vi "Test Packet Identifier.vi"() -> ()   [LabVIEW 2013]
uses:
  Control Packets/CONNECT/CONNECT.lvclass
  Control Packets/CONNACK/CONNACK.lvclass
  Control Packets/PUBLISH/PUBLISH.lvclass
  Control Packets/PUBACK/PUBACK.lvclass
  Control Packets/PUBREC/PUBREC.lvclass
  Control Packets/PUBREL/PUBREL.lvclass
  Control Packets/PUBCOMP/PUBCOMP.lvclass
  Control Packets/SUBSCRIBE/SUBSCRIBE.lvclass
  Control Packets/SUBACK/SUBACK.lvclass
  Control Packets/UNSUBSCRIBE/UNSUBSCRIBE.lvclass
  Control Packets/UNSUBACK/UNSUBACK.lvclass
  Control Packets/PINGREC/PINGREC.lvclass
  Control Packets/PINGRESP/PINGRESP.lvclass
  Control Packets/DISCONNECT/DISCONNECT.lvclass
  Control Packets/ControlPacket/ControlPacket.lvclass/ControlPacket.ctl
  Control Packets/ControlPacket/ControlPacket.lvclass
panel:
  out "PASS":bool
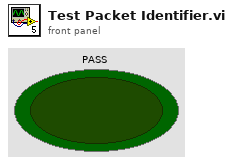
[diagram p1: front panel]
types:
  T1 = cluster{"CONNECT":refnum<class "CONNECT.lvclass">, "CONNACK":refnum<class "CONNACK.lvclass">, "PUBLISH":refnum<class "PUBLISH.lvclass">, "PUBACK":refnum<class "PUBACK.lvclass">, "PUBREC":refnum<class "PUBREC.lvclass">, "PUBREL":refnum<class "PUBREL.lvclass">, "PUBCOMP":refnum<class "PUBCOMP.lvclass">, "SUBSCRIBE":refnum<class "SUBSCRIBE.lvclass">, "SUBACK":refnum<class "SUBACK.lvclass">, "UNSUBSCRIBE":refnum<class "UNSUBSCRIBE.lvclass">, "UNSUBACK":refnum<class "UNSUBACK.lvclass">, "PINGREC":refnum<class "PINGREC.lvclass">, "PINGRESP":refnum<class "PINGRESP.lvclass">, "DISCONNECT":refnum<class "DISCONNECT.lvclass">}
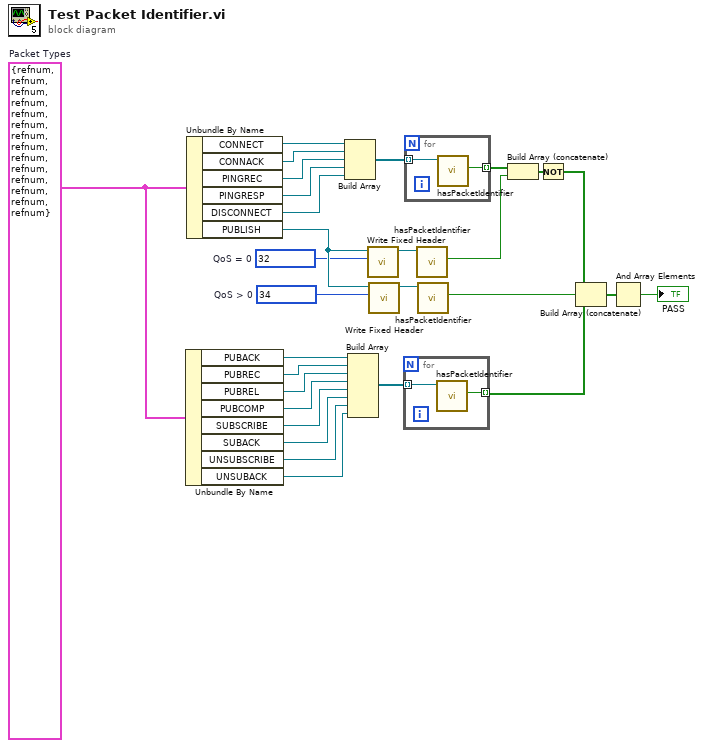
[diagram p0: block diagram]
diagram:
  w1 = u8 32  # QoS = 0
  w11 = u8 34  # QoS > 0
  w29 = T1 {"CONNECT"=refnum, "CONNACK"=refnum, "PUBLISH"=refnum, "PUBACK"=refnum, "PUBREC"=refnum, "PUBREL"=refnum, "PUBCOMP"=refnum, "SUBSCRIBE"=refnum, "SUBACK"=refnum, "UNSUBSCRIBE"=refnum, "UNSUBACK"=refnum, "PINGREC"=refnum, "PINGRESP"=refnum, "DISCONNECT"=refnum}  # Packet Types
  n1 = Unbundle By Name(w29) -> ("PUBACK"=w23:refnum<class "PUBACK.lvclass">, "PUBREC"=w22:refnum<class "PUBREC.lvclass">, "PUBREL"=w21:refnum<class "PUBREL.lvclass">, "PUBCOMP"=w20:refnum<class "PUBCOMP.lvclass">, "SUBSCRIBE"=w19:refnum<class "SUBSCRIBE.lvclass">, "SUBACK"=w18:refnum<class "SUBACK.lvclass">, "UNSUBSCRIBE"=w17:refnum<class "UNSUBSCRIBE.lvclass">, "UNSUBACK"=w16:refnum<class "UNSUBACK.lvclass">)
  n2 = Unbundle By Name(w29) -> ("CONNECT"=w28:refnum<class "CONNECT.lvclass">, "CONNACK"=w27:refnum<class "CONNACK.lvclass">, "PINGREC"=w26:refnum<class "PINGREC.lvclass">, "PINGRESP"=w25:refnum<class "PINGRESP.lvclass">, "DISCONNECT"=w24:refnum<class "DISCONNECT.lvclass">, "PUBLISH"=w3:refnum<class "PUBLISH.lvclass">)
  n3 = Build Array(w28, w27, w26, w25, w24) -> (w15:refnum<class "ControlPacket.lvclass">[])
  n4 = Build Array(w23, w22, w21, w20, w19, w18, w17, w16) -> (w14:refnum<class "ControlPacket.lvclass">[])
  n5 = call "Write Fixed Header.vi"("Fixed Header"=w1, "ControlPacket in"=w3) -> ("ControlPacket out"=w2:refnum<class "PUBLISH.lvclass">)  [unwired: 9 in]
  n6 = call "Write Fixed Header.vi"("Fixed Header"=w11, "ControlPacket in"=w3) -> ("ControlPacket out"=w10:refnum<class "PUBLISH.lvclass">)  [unwired: 9 in]
  n7 = for {
    tunnel: w14 -> [w31] mode=indexing
    tunnel: [w30] -> w8 mode=indexing
    n8 = call-dynamic "hasPacketIdentifier.vi"("ControlPacket in"=w31) -> ("As Packet Identifier"=w30:bool)  [unwired: 9 in, 1 out]
  }
  n9 = for {
    tunnel: w15 -> [w33] mode=indexing
    tunnel: [w32] -> w7 mode=indexing
    n10 = call-dynamic "hasPacketIdentifier.vi"("ControlPacket in"=w33) -> ("As Packet Identifier"=w32:bool)  [unwired: 9 in, 1 out]
  }
  n11 = call-dynamic "hasPacketIdentifier.vi"("PUBLISH in"=w2) -> ("As Packet Identifier"=w6:bool)  [unwired: 9 in, 1 out]
  n12 = call-dynamic "hasPacketIdentifier.vi"("PUBLISH in"=w10) -> ("As Packet Identifier"=w9:bool)  [unwired: 9 in, 1 out]
  n13 = Build Array (concatenate)(w7, w6) -> (w5:bool[])
  n14 = Not(x=w5) -> (.not. x?=w4:bool[])
  n15 = Build Array (concatenate)(w4, w9, w8) -> (w13:bool[])
  n16 = And Array Elements(Boolean array=w13) -> (logical AND=→"PASS":bool)
